vi "Set TableName.vi"(8 "error in (no error)":errorcluster, 10 "TableName":string, 11 "ScriptDatabase in":refnum<class "ScriptDatabase.lvclass">) -> (0 "error out":errorcluster, 3 "ScriptDatabase out":refnum<class "ScriptDatabase.lvclass">)   [LabVIEW 2015, in "ScriptDatabase.lvclass"]
uses:
  ScriptDatabase.lvclass
  ScriptDatabase.lvclass/ScriptDatabase.ctl
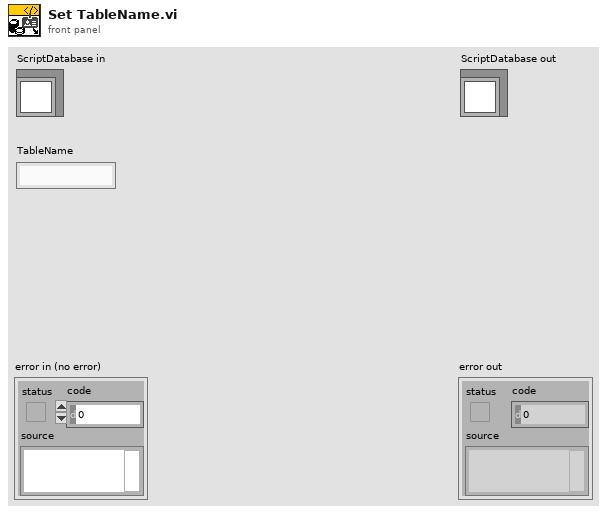
[diagram p1: front panel]
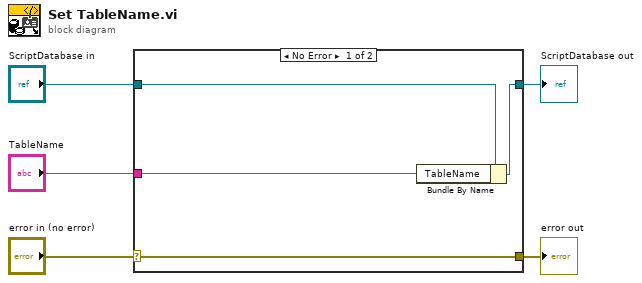
[diagram p0: block diagram]
diagram:
  n1 = case shown="No Error" "error in (no error)" {
    selector: "error in (no error)" -> [w9 w10]
    tunnel: [w9 w10] -> w4
    tunnel: [w7 w11] -> w2
    tunnel: "ScriptDatabase in" -> [w8 w11]
    tunnel: "TableName" -> [w6 _]
    frame No Error {
      n2 = Bundle By Name(cluster=w8, "TableName"=w6) -> (w7:refnum<class "ScriptDatabase.lvclass">)
    }
    frame Error {
    }
  }
  "error out" <- w4
  "ScriptDatabase out" <- w2
